vi "Obtain Default Broadcast Events.vi"(8 "error in (no error)":errorcluster) -> (0 "error out":errorcluster, 1 "Update Module Execution Status":refnum<user-event>, 2 "Error Reported":refnum<user-event>, 3 "Status Updated":refnum<user-event>, 4 "System Message":refnum<user-event>, 5 "Module Did Stop":refnum<user-event>)   [LabVIEW 2022 SP3, in "ExampleClone.lvlib"]
doc: "____\nHAMPEL SOFTWARE ENGINEERING v2.6.0 (2023-12-19 10:54)"
uses:
  ExampleClone.lvlib
  Status Updated Argument--cluster.ctl
  Error Reported Argument--cluster.ctl
  Stop Argument--cluster.ctl
  Get Module Execution Status Argument--cluster.ctl
  System Message Argument--cluster.ctl
  Libraries/hse-libraries/Source/hse-dqmh/Controls/System Message Source.ctl
  Libraries/hse-libraries/Source/hse-dqmh/hse-dqmh.lvlib
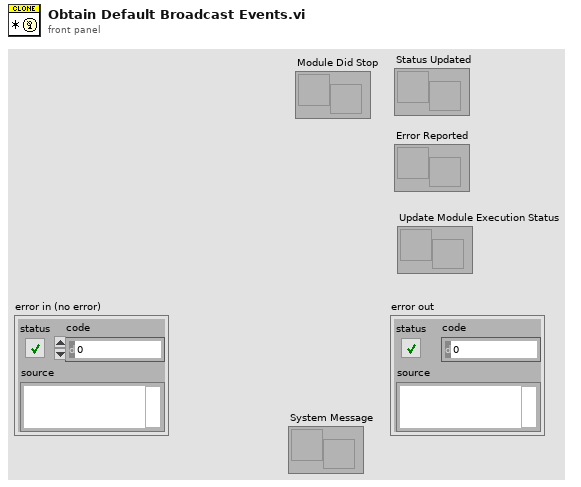
[diagram p1: front panel]
types:
  T1 = typedef "ExampleClone.lvlib/Broadcast Events--cluster.ctl" = cluster{"Module Did Init":refnum<user-event>, "Status Updated":refnum<user-event>, "Error Reported":refnum<user-event>, "Module Did Stop":refnum<user-event>, "Update Module Execution Status":refnum<user-event>, "System Message":refnum<user-event>}
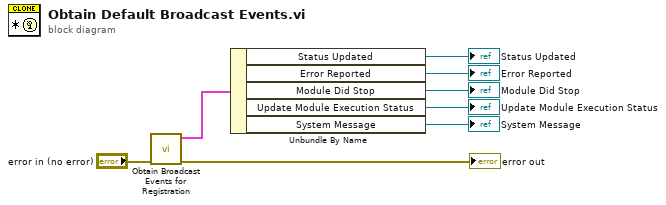
[diagram p0: block diagram]
diagram:
  n1 = call "Obtain Broadcast Events for Registration.vi"("error in (no error)"="error in (no error)") -> ("error out"=→"error out":errorcluster, "ExampleClone Broadcast Events"=w6:T1)  [unwired: 9 in]
  n2 = Unbundle By Name(w6) -> ("Status Updated"=→"Status Updated":refnum<user-event>, "Error Reported"=→"Error Reported":refnum<user-event>, "Module Did Stop"=→"Module Did Stop":refnum<user-event>, "Update Module Execution Status"=→"Update Module Execution Status":refnum<user-event>, "System Message"=→"System Message":refnum<user-event>)
